vi "ID Pool Error Info.vi"(11 "error":T1) -> (3 "error info":cluster{"code":i32, "description":string})   [LabVIEW 2017, in "DSF Core.lvlib" / "ID Pool.lvclass"]
uses:
  ID Pool.lvclass
  Errors.ctl
  VIs/Constants/Base Error Code.vi
  DSF Core.lvlib
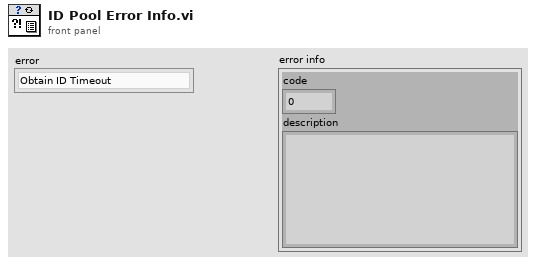
[diagram p1: front panel]
types:
  T1 = typedef "DSF Core.lvlib/ID Pool.lvclass/Errors.ctl" = enum16{"Obtain ID Timeout", "Return ID Timeout"}
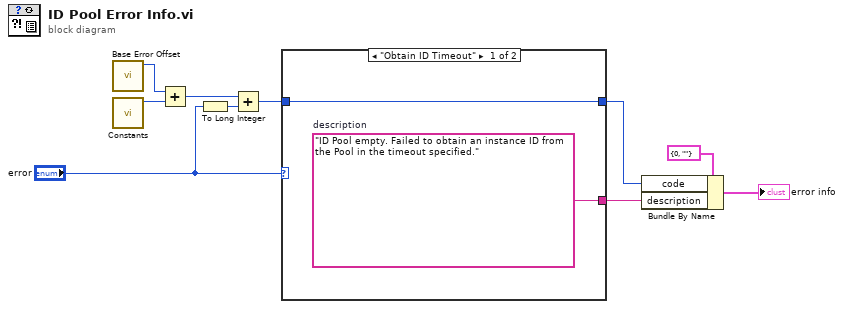
[diagram p0: block diagram]
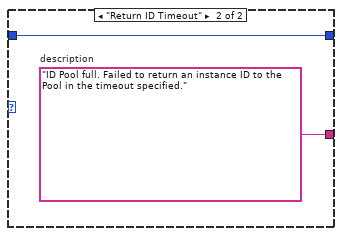
[diagram p2: hidden frame]
diagram:
  n1 = call "Base Error Offset.vi"() -> ("base error offset"=w2:i32)  [unwired: 11 in]
  n2 = call-poly "Constants.vi"() -> ("base error code"=w10:i32)  [unwired: 11 in]
  n3 = Add(x=w2, y=w10) -> (x+y=w6:i32)
  n4 = To Long Integer(number="error") -> (32bit integer=w9:i32)
  n5 = Add(x=w6, y=w9) -> (x+y=w5:i32)
  n6 = case shown="\"Obtain ID Timeout\"" "error" {
    tunnel: [w12 w14] -> w7
    tunnel: w5 -> [w11 w13]
    tunnel: [w11 w13] -> w4
    frame "Obtain ID Timeout" {
      w12 = "ID Pool empty. Failed to obtain an instance ID from the Pool in the timeout specified."  # description
    }
    frame "Return ID Timeout" {
      w14 = "ID Pool full. Failed to return an instance ID to the Pool in the timeout specified."  # description
    }
  }
  n7 = Bundle By Name(cluster=cluster{"code":i32, "description":string} {"code"=0, "description"=""}, "code"=w4, "description"=w7) -> (→"error info":cluster{"code":i32, "description":string})
